vi "CfgFile Set Desc Frame Basic.vi"(8 "error in (no error)":errorcluster, 9 "Frame Skill":T1, 10 "Frame Basic":T3, 11 "LF2R IDE in":refnum<class "LF2R IDE.lvclass">) -> (0 "error out":errorcluster, 3 "LF2R IDE out":refnum<class "LF2R IDE.lvclass">)   [LabVIEW 2018, in "LF2R IDE.lvlib" / "LF2R IDE.lvclass"]
uses:
  LF2R IDE.lvclass
  Const UI Desc Frame Basic.ctl
  Const UI Property.ctl
  Const UI Desc Frame Skill.ctl
  LF2R IDE.lvclass/LF2R IDE.ctl
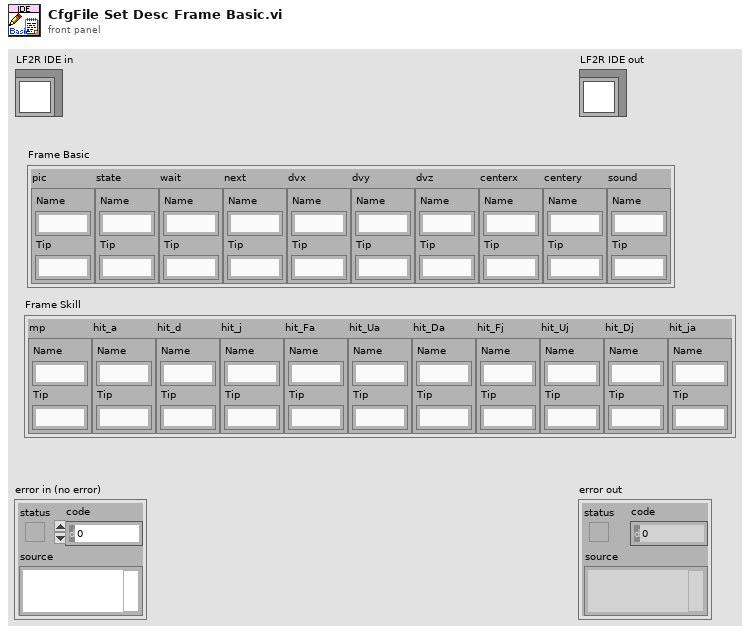
[diagram p1: front panel]
types:
  T1 = typedef "LF2R IDE.lvlib/LF2R IDE.lvclass/Const UI Desc Frame Skill.ctl" = cluster{"mp":T2, "hit_a":T2, "hit_d":T2, "hit_j":T2, "hit_Fa":T2, "hit_Ua":T2, "hit_Da":T2, "hit_Fj":T2, "hit_Uj":T2, "hit_Dj":T2, "hit_ja":T2}
  T2 = typedef "LF2R IDE.lvlib/LF2R IDE.lvclass/Const UI Property.ctl" = cluster{"Name":string, "Tip":string}
  T3 = typedef "LF2R IDE.lvlib/LF2R IDE.lvclass/Const UI Desc Frame Basic.ctl" = cluster{"pic":T2, "state":T2, "wait":T2, "next":T2, "dvx":T2, "dvy":T2, "dvz":T2, "centerx":T2, "centery":T2, "sound":T2}
  T4 = cluster{"pic":refnum<vi>, "state":refnum<vi>, "wait":refnum<vi>, "next":refnum<vi>}
  T5 = cluster{"dvx":refnum<vi>, "dvy":refnum<vi>, "dvz":refnum<vi>}
  T6 = cluster{"centerx":refnum<vi>, "centery":refnum<vi>}
  T7 = cluster{"hit_a":refnum<vi>, "hit_d":refnum<vi>, "hit_j":refnum<vi>, "hit_Fa":refnum<vi>, "hit_Ua":refnum<vi>, "hit_Da":refnum<vi>, "hit_Fj":refnum<vi>, "hit_Uj":refnum<vi>, "hit_Dj":refnum<vi>, "hit_ja":refnum<vi>}
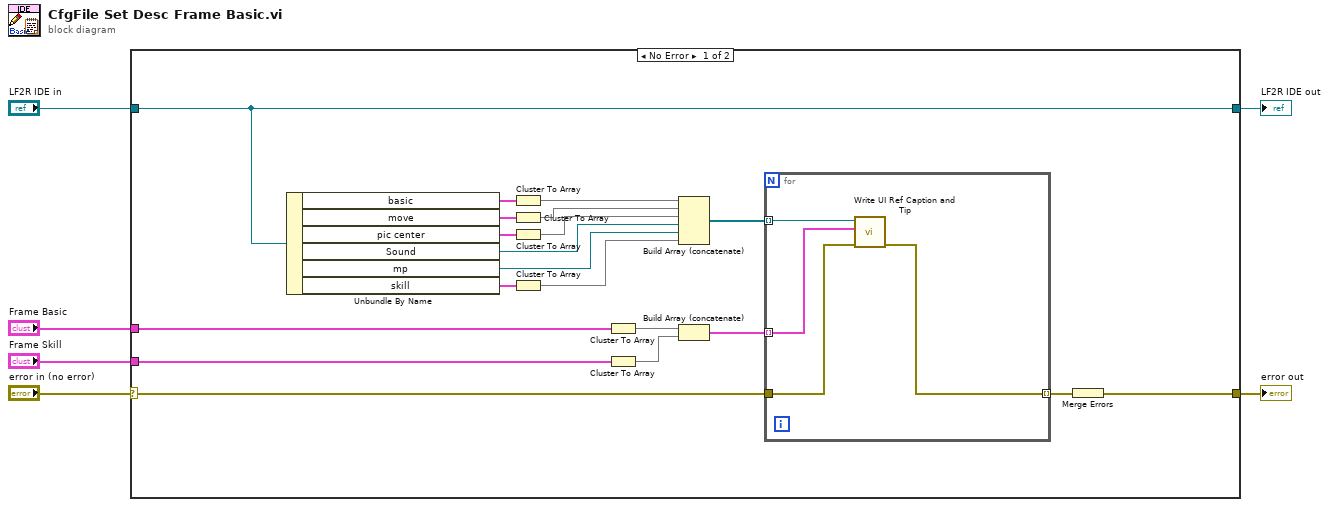
[diagram p0: block diagram]
diagram:
  n1 = case shown="No Error" "error in (no error)" {
    selector: "error in (no error)" -> [w10 w32]
    tunnel: [w8 w32] -> w5
    tunnel: [w26 w31] -> w3
    tunnel: "LF2R IDE in" -> [w26 w31]
    tunnel: "Frame Basic" -> [w15 _]
    tunnel: "Frame Skill" -> [w14 _]
    frame No Error {
      n2 = Unbundle By Name(w26) -> ("basic"=w25:T4, "move"=w24:T5, "pic center"=w22:T6, "Sound"=w7:refnum<vi>, "mp"=w18:refnum<vi>, "skill"=w23:T7)
      n3 = Cluster To Array(cluster=w25) -> (array=w21:refnum<vi>[])
      n4 = Cluster To Array(cluster=w24) -> (array=w20:refnum<vi>[])
      n5 = Cluster To Array(cluster=w22) -> (array=w19:refnum<vi>[])
      n6 = Cluster To Array(cluster=w23) -> (array=w17:refnum<vi>[])
      n7 = Cluster To Array(cluster=w15) -> (array=w13:T2[])
      n8 = Cluster To Array(cluster=w14) -> (array=w12:T2[])
      n9 = Build Array (concatenate)(w21, w20, w19, w7, w18, w17) -> (w16:refnum<vi>[])
      n10 = Build Array (concatenate)(w13, w12) -> (w11:T2[])
      n11 = for {
        tunnel: w16 -> [w30] mode=indexing
        tunnel: w11 -> [w29] mode=indexing
        tunnel: w10 -> [w28]
        tunnel: [w27] -> w9 mode=indexing
        n12 = call "Write UI Ref Caption and Tip.vi"("error in (no error)"=w28, "UI Property"=w29, "UI Ref"=w30) -> ("error out"=w27:errorcluster)  [unwired: 8 in]
      }
      n13 = Merge Errors(w9) -> (w8:errorcluster)
    }
    frame Error {
    }
  }
  "error out" <- w5
  "LF2R IDE out" <- w3
